vi "Longest Completion Time Job MO Swap.vi"(8 "error in (no error)":errorcluster, 9 "Schedule in":u16[](array[numeric]), 10 "OSSP_Problem":refnum<class "OSSP_Problem.lvclass">, 11 "GA in":refnum<class "GA.lvclass">) -> (0 "error out":errorcluster, 1 "Schedule out":u16[](array[numeric]), 2 "OSSP_Problem out":refnum<class "OSSP_Problem.lvclass">, 3 "GA out":refnum<class "GA.lvclass">)   [LabVIEW 2013, in "GA.lvclass"]
uses:
  GA.lvclass
  OSSP_Problem.lvclass
  GA.lvclass/GA.ctl
  OSSP_Problem.lvclass/OSSP_Problem.ctl
  Scheduler_Class/Operation to Machine Job Tuple.vi
  Scheduler_Class/Check Other Machines for Schedule Time.vi
  Scheduler_Class/Schedule Job.vi
  Scheduler_Class/Find Gaps on Particular Machine.vi
  Scheduler_Class/Increment Number of Jobs on Machine.vi
  Scheduler_Class/Find Job On Other Machines.vi
  Scheduler_Class/Prins FIFO Scheduler Methods and Controls/Methods/UpdateMachineGaps.vi
  Scheduler_Class/Prins FIFO Scheduler Methods and Controls/Methods/UpdateJobGaps.vi
  Scheduler_Class/Prins FIFO Scheduler Methods and Controls/Methods/Find Intersecting Gaps.vi
  Scheduler_Class/GT Algorithm Find M_ok and J_ok.vi
  Scheduler_Class/Prins FIFO Scheduler Methods and Controls/Methods/Transform to Plain Job and Machine Gaps Array.vi
  Scheduler.lvclass
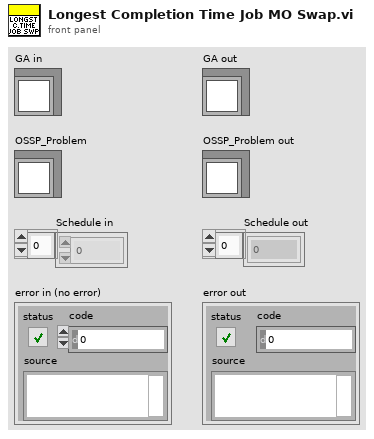
[diagram p1: front panel]
types:
  T1 = typedef "Objective.ctl" = enum16{"Makespan", "Total Tardiness"}
  T2 = typedef "Scheduler Type.ctl" = enum16{"Non Delay Scheduler", "GT Active Scheduler", "My Faulty Scheduler", "Prins FIFO Scheduler", "SemiActive Scheduler"}
  T3 = typedef "GanntChart_Element.ctl" = cluster{"Operation Number":i32, "Job Number":i32, "Start Time":i32, "Procesing Time":u16, "End Time":i32}
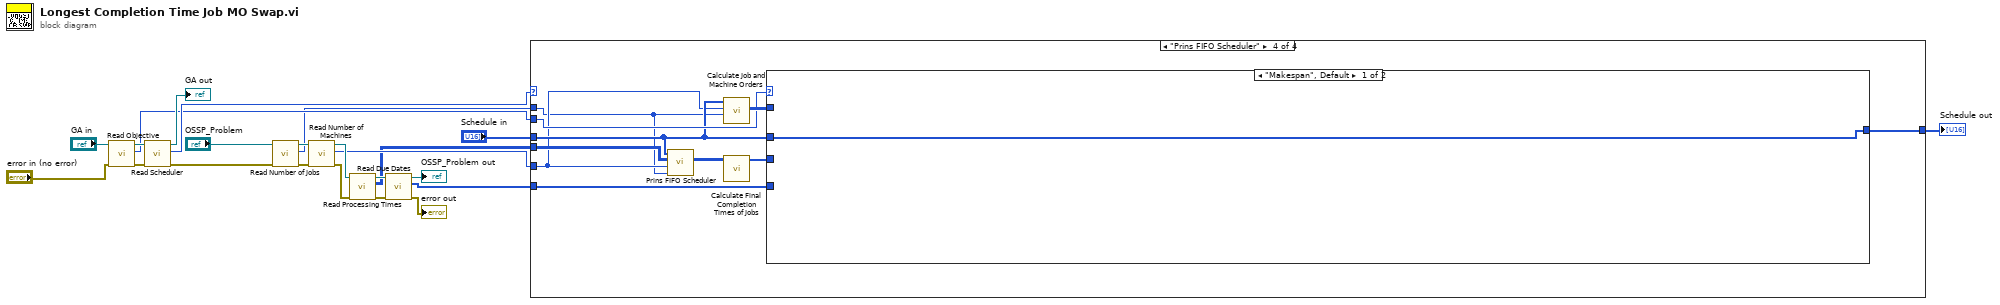
[diagram p0: block diagram]
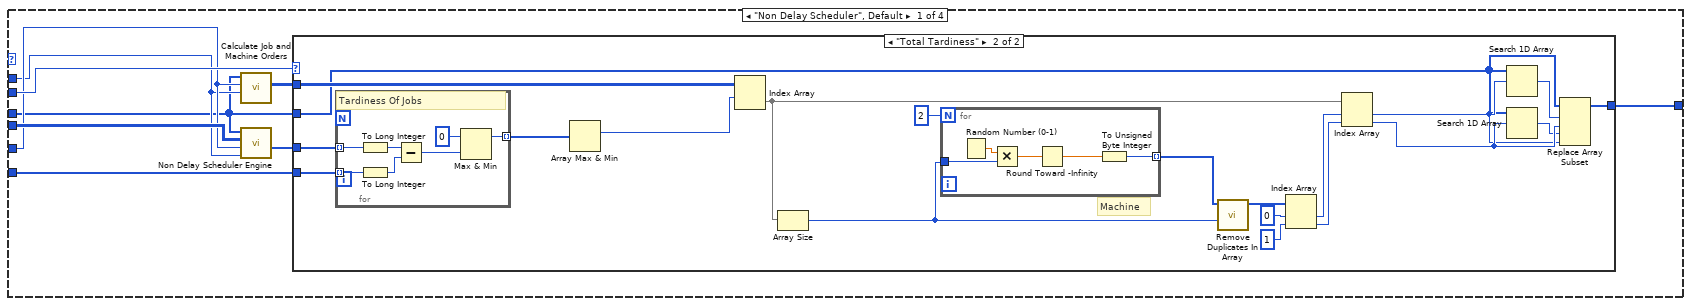
[diagram p2: hidden frame]
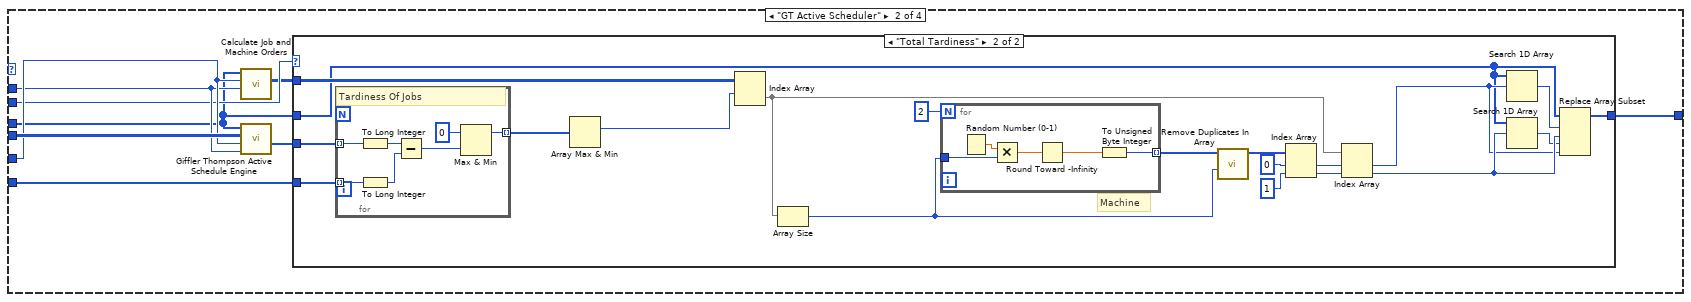
[diagram p4: hidden frame]
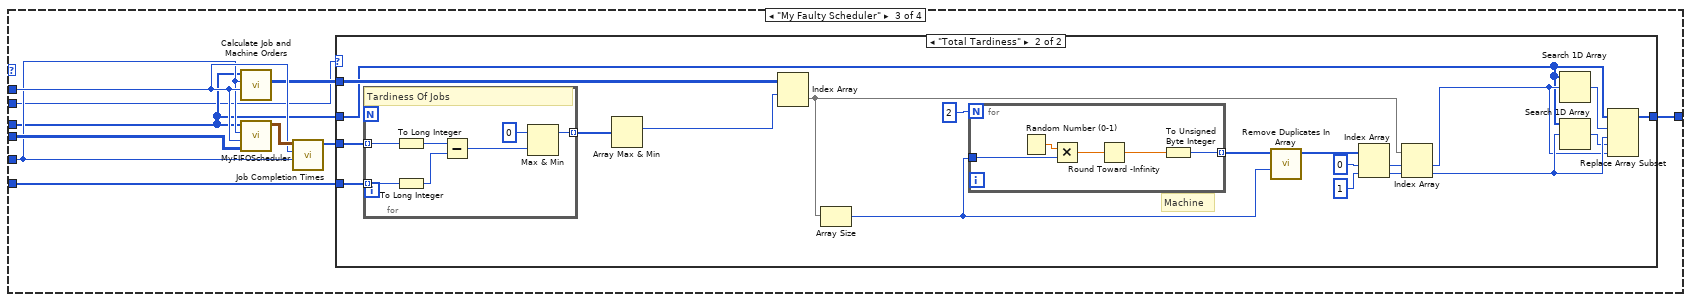
[diagram p6: hidden frame]
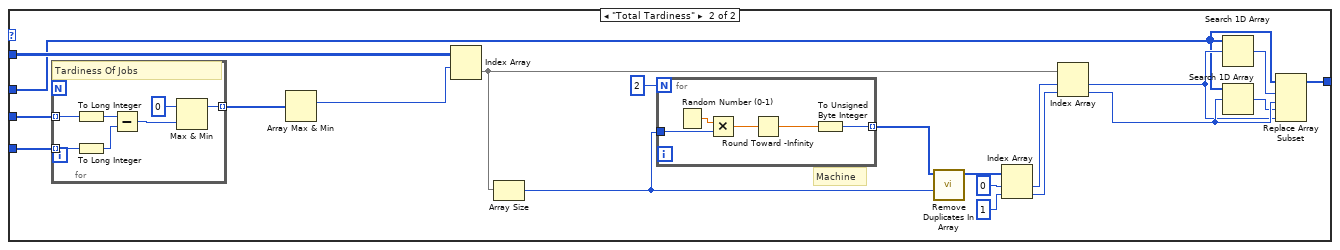
[diagram p8: hidden frame]
diagram:
  n1 = call "Read Objective .vi"("error in (no error)"="error in (no error)", "GA in"="GA in") -> ("error out"=w14:errorcluster, "Objective"=w12:T1, "GA out"=w15:refnum<class "GA.lvclass">)  [unwired: 7 in]
  n2 = call "Read Scheduler.vi"("error in (no error)"=w14, "GA in"=w15) -> ("error out"=w5:errorcluster, "Scheduler"=w13:T2, "GA out"=→"GA out":refnum<class "GA.lvclass">)  [unwired: 7 in]
  n3 = call "Read Number of Jobs.vi"("error in (no error)"=w5, "OSSP_Problem in"="OSSP_Problem") -> ("error out"=w8:errorcluster, "Number of Jobs"=w4:i32, "OSSP_Problem out"=w11:refnum<class "OSSP_Problem.lvclass">)  [unwired: 7 in]
  n4 = call "Read Number of Machines.vi"("error in (no error)"=w8, "OSSP_Problem in"=w11) -> ("error out"=w7:errorcluster, "Number of Machines"=w3:i32, "OSSP_Problem out"=w10:refnum<class "OSSP_Problem.lvclass">)  [unwired: 7 in]
  n5 = call "Read Processing Times.vi"("error in (no error)"=w7, "OSSP_Problem in"=w10) -> ("error out"=w6:errorcluster, "Processing Times"=w2:u16[][], "OSSP_Problem out"=w9:refnum<class "OSSP_Problem.lvclass">)  [unwired: 7 in]
  n6 = call "Read Due Dates.vi"("error in (no error)"=w6, "OSSP_Problem in"=w9) -> ("error out"=→"error out":errorcluster, "Due Dates"=w1:u16[], "OSSP_Problem out"=→"OSSP_Problem out":refnum<class "OSSP_Problem.lvclass">)  [unwired: 7 in]
  n7 = case shown="\"Prins FIFO Scheduler\"" w13 {
    tunnel: w12 -> [w32 w69 w108 w157]
    tunnel: w4 -> [w28 w72 w115 w153]
    tunnel: w3 -> [w29 w73 w114 w154]
    tunnel: w2 -> [w31 w74 w116 w155]
    tunnel: w1 -> [w26 w70 w112 w160]
    tunnel: "Schedule in" -> [w25 w66 w110 w156]
    tunnel: [w24 w67 w109 w158] -> w23
    frame "Non Delay Scheduler", Default {
      n8 = call "Calculate Job and Machine Orders.vi"("Number of Jobs"=w28, "Number of Machines"=w29, "Schedule"=w25) -> ("MO4J"=w27:u16[][])  [unwired: 7 in, 1 out]
      n9 = call "Non Delay Scheduler Engine.vi"("Number of  Jobs"=w28, "Number of Machines"=w29, "Processing Times"=w31, "Schedule"=w25) -> ("Job Completion Times"=w30:u16[])  [unwired: 2 in, 5 out]
      n10 = case shown="\"Total Tardiness\"" w32 {
        tunnel: w30 -> [_ w53]
        tunnel: w27 -> [_ w50]
        tunnel: w26 -> [_ w52]
        tunnel: w25 -> [w33 w35]
        tunnel: [w33 w34] -> w24
        frame "Makespan", Default {
        }
        frame "Total Tardiness" {
          # "Machine"
          n11 = for {
            tunnel: w53 -> [w65] mode=indexing
            tunnel: w52 -> [w64] mode=indexing
            tunnel: [w59] -> w51 mode=indexing
            # "Tardiness Of Jobs"
            n12 = To Long Integer(number=w65) -> (32bit integer=w63:i32)
            n13 = To Long Integer(number=w64) -> (32bit integer=w62:i32)
            n14 = Subtract(x=w63, y=w62) -> (x-y=w61:i32)
            n15 = Max & Min(x=0, y=w61) -> (max(x,y)=w59:i32)  [unwired: 1 out]
          }
          n16 = Array Max & Min(array=w51) -> (max index (indices)=w49:i32)  [unwired: 3 out]
          n17 = Index Array(array=w50, index (row)=w49) -> (element=w37:u16[])  [unwired: 1 in]
          n18 = Array Size(array=w37) -> (size(s)=w38:i32)
          n19 = for {
            N: 2 -> [_]
            tunnel: w38 -> [w57]
            tunnel: [w54] -> w41 mode=indexing
            n20 = Random Number (0-1)() -> (number: 0 to 1=w58:dbl)
            n21 = Multiply(x=w58, y=w57) -> (x*y=w56:dbl)
            n22 = Round Toward -Infinity(1:w56) -> (0:w55:dbl)
            n23 = To Unsigned Byte Integer(number=w55) -> (unsigned 8bit integer=w54:u8)
          }
          n24 = call "Remove Duplicates In Array.vi"("Max Index Bound"=w38, "Random Numbers Array"=w41) -> ("Random Numbers Array without Duplicates"=w39:i32[])  [unwired: 9 in]
          n25 = Index Array(array=w39, index #1=0 ("index"), index #2=1 ("index")) -> (element #1=w46:i32, element #2=w45:i32)
          n26 = Index Array(array=w37, index #1=w46, index #2=w45) -> (element #1=w36:u16, element #2=w43:u16)
          n27 = Search 1D Array(1D array=w35, element=w36) -> (index of element=w44:i32)  [unwired: 1 in]
          n28 = Search 1D Array(1D array=w35, element=w43) -> (index of element=w42:i32)  [unwired: 1 in]
          n29 = Replace Array Subset(array=w35, new element #1=w43, index #1=w44, new element #2=w36, index #2=w42) -> (w34:u16[])
        }
      }
    }
    frame "GT Active Scheduler" {
      n30 = call "Calculate Job and Machine Orders.vi"("Number of Jobs"=w72, "Number of Machines"=w73, "Schedule"=w66) -> ("MO4J"=w68:u16[][])  [unwired: 7 in, 1 out]
      n31 = call "Giffler Thompson Active Schedule Engine.vi"("Number of  Jobs"=w72, "Number of Machines"=w73, "Processing Times"=w74, "Schedule In"=w66) -> ("Job Completion Times"=w71:u16[])  [unwired: 3 in, 4 out]
      n32 = case shown="\"Total Tardiness\"" w69 {
        tunnel: w71 -> [_ w95]
        tunnel: w68 -> [_ w92]
        tunnel: w70 -> [_ w94]
        tunnel: w66 -> [w75 w77]
        tunnel: [w75 w76] -> w67
        frame "Makespan", Default {
        }
        frame "Total Tardiness" {
          # "Machine"
          n33 = for {
            tunnel: w95 -> [w107] mode=indexing
            tunnel: w94 -> [w106] mode=indexing
            tunnel: [w101] -> w93 mode=indexing
            # "Tardiness Of Jobs"
            n34 = To Long Integer(number=w107) -> (32bit integer=w105:i32)
            n35 = To Long Integer(number=w106) -> (32bit integer=w104:i32)
            n36 = Subtract(x=w105, y=w104) -> (x-y=w103:i32)
            n37 = Max & Min(x=0, y=w103) -> (max(x,y)=w101:i32)  [unwired: 1 out]
          }
          n38 = Array Max & Min(array=w93) -> (max index (indices)=w91:i32)  [unwired: 3 out]
          n39 = Index Array(array=w92, index (row)=w91) -> (element=w79:u16[])  [unwired: 1 in]
          n40 = Array Size(array=w79) -> (size(s)=w80:i32)
          n41 = for {
            N: 2 -> [_]
            tunnel: w80 -> [w99]
            tunnel: [w96] -> w83 mode=indexing
            n42 = Random Number (0-1)() -> (number: 0 to 1=w100:dbl)
            n43 = Multiply(x=w100, y=w99) -> (x*y=w98:dbl)
            n44 = Round Toward -Infinity(1:w98) -> (0:w97:dbl)
            n45 = To Unsigned Byte Integer(number=w97) -> (unsigned 8bit integer=w96:u8)
          }
          n46 = call "Remove Duplicates In Array.vi"("Max Index Bound"=w80, "Random Numbers Array"=w83) -> ("Random Numbers Array without Duplicates"=w81:i32[])  [unwired: 9 in]
          n47 = Index Array(array=w81, index #1=0 ("index"), index #2=1 ("index")) -> (element #1=w88:i32, element #2=w87:i32)
          n48 = Index Array(array=w79, index #1=w88, index #2=w87) -> (element #1=w78:u16, element #2=w85:u16)
          n49 = Search 1D Array(1D array=w77, element=w78) -> (index of element=w86:i32)  [unwired: 1 in]
          n50 = Search 1D Array(1D array=w77, element=w85) -> (index of element=w84:i32)  [unwired: 1 in]
          n51 = Replace Array Subset(array=w77, new element #1=w85, index #1=w86, new element #2=w78, index #2=w84) -> (w76:u16[])
        }
      }
    }
    frame "My Faulty Scheduler" {
      n52 = call "Calculate Job and Machine Orders.vi"("Number of Jobs"=w115, "Number of Machines"=w114, "Schedule"=w110) -> ("MO4J"=w111:u16[][])  [unwired: 7 in, 1 out]
      n53 = call "MyFIFOScheduler.vi"("Processing Times (Rows Mach.Cols Jobs)"=w116, "Number of Jobs"=w115, "Number of Machines"=w114, "Schedule"=w110) -> ("Gannt Chart Out"=w117:T3[][])  [unwired: 6 in, 1 out]
      n54 = call "Job Completion Times.vi"("Number Of Machines"=w114, "Number Of Jobs"=w115, "Gannt Chart In"=w117) -> ("Job Completion Times"=w113:u16[])  [unwired: 8 in]
      n55 = case shown="\"Total Tardiness\"" w108 {
        tunnel: w113 -> [_ w138]
        tunnel: w111 -> [_ w135]
        tunnel: w112 -> [_ w137]
        tunnel: w110 -> [w118 w120]
        tunnel: [w118 w119] -> w109
        frame "Makespan", Default {
        }
        frame "Total Tardiness" {
          # "Machine"
          n56 = for {
            tunnel: w138 -> [w150] mode=indexing
            tunnel: w137 -> [w149] mode=indexing
            tunnel: [w144] -> w136 mode=indexing
            # "Tardiness Of Jobs"
            n57 = To Long Integer(number=w150) -> (32bit integer=w148:i32)
            n58 = To Long Integer(number=w149) -> (32bit integer=w147:i32)
            n59 = Subtract(x=w148, y=w147) -> (x-y=w146:i32)
            n60 = Max & Min(x=0, y=w146) -> (max(x,y)=w144:i32)  [unwired: 1 out]
          }
          n61 = Array Max & Min(array=w136) -> (max index (indices)=w134:i32)  [unwired: 3 out]
          n62 = Index Array(array=w135, index (row)=w134) -> (element=w122:u16[])  [unwired: 1 in]
          n63 = Array Size(array=w122) -> (size(s)=w123:i32)
          n64 = for {
            N: 2 -> [_]
            tunnel: w123 -> [w142]
            tunnel: [w139] -> w126 mode=indexing
            n65 = Random Number (0-1)() -> (number: 0 to 1=w143:dbl)
            n66 = Multiply(x=w143, y=w142) -> (x*y=w141:dbl)
            n67 = Round Toward -Infinity(1:w141) -> (0:w140:dbl)
            n68 = To Unsigned Byte Integer(number=w140) -> (unsigned 8bit integer=w139:u8)
          }
          n69 = call "Remove Duplicates In Array.vi"("Max Index Bound"=w123, "Random Numbers Array"=w126) -> ("Random Numbers Array without Duplicates"=w124:i32[])  [unwired: 9 in]
          n70 = Index Array(array=w124, index #1=0 ("index"), index #2=1 ("index")) -> (element #1=w131:i32, element #2=w130:i32)
          n71 = Index Array(array=w122, index #1=w131, index #2=w130) -> (element #1=w121:u16, element #2=w128:u16)
          n72 = Search 1D Array(1D array=w120, element=w121) -> (index of element=w129:i32)  [unwired: 1 in]
          n73 = Search 1D Array(1D array=w120, element=w128) -> (index of element=w127:i32)  [unwired: 1 in]
          n74 = Replace Array Subset(array=w120, new element #1=w128, index #1=w129, new element #2=w121, index #2=w127) -> (w119:u16[])
        }
      }
    }
    frame "Prins FIFO Scheduler" {
      n75 = call "Prins FIFO Scheduler.vi"("Number of Jobs"=w153, "Number of Machines"=w154, "Processing Times(MxJ)"=w155, "Schedule In"=w156) -> ("Completion Times (MxJ)"=w152:i32[][])  [unwired: 6 in, 1 out]
      n76 = call "Calculate Job and Machine Orders.vi"("Number of Jobs"=w153, "Number of Machines"=w154, "Schedule"=w156) -> ("MO4J"=w159:u16[][])  [unwired: 7 in, 1 out]
      n77 = call "Calculate Final Completion Times of Jobs.vi"("Completion Times (MxJ)"=w152) -> ("Job Completion Times"=w151:i32[])  [unwired: 10 in]
      n78 = case shown="\"Makespan\", Default" w157 {
        tunnel: w151 -> [_ w181]
        tunnel: w159 -> [_ w178]
        tunnel: w160 -> [_ w180]
        tunnel: w156 -> [w161 w163]
        tunnel: [w161 w162] -> w158
        frame "Makespan", Default {
        }
        frame "Total Tardiness" {
          # "Machine"
          n79 = for {
            tunnel: w181 -> [w193] mode=indexing
            tunnel: w180 -> [w192] mode=indexing
            tunnel: [w187] -> w179 mode=indexing
            # "Tardiness Of Jobs"
            n80 = To Long Integer(number=w193) -> (32bit integer=w191:i32)
            n81 = To Long Integer(number=w192) -> (32bit integer=w190:i32)
            n82 = Subtract(x=w191, y=w190) -> (x-y=w189:i32)
            n83 = Max & Min(x=0, y=w189) -> (max(x,y)=w187:i32)  [unwired: 1 out]
          }
          n84 = Array Max & Min(array=w179) -> (max index (indices)=w177:i32)  [unwired: 3 out]
          n85 = Index Array(array=w178, index (row)=w177) -> (element=w165:u16[])  [unwired: 1 in]
          n86 = Array Size(array=w165) -> (size(s)=w166:i32)
          n87 = for {
            N: 2 -> [_]
            tunnel: w166 -> [w185]
            tunnel: [w182] -> w169 mode=indexing
            n88 = Random Number (0-1)() -> (number: 0 to 1=w186:dbl)
            n89 = Multiply(x=w186, y=w185) -> (x*y=w184:dbl)
            n90 = Round Toward -Infinity(1:w184) -> (0:w183:dbl)
            n91 = To Unsigned Byte Integer(number=w183) -> (unsigned 8bit integer=w182:u8)
          }
          n92 = call "Remove Duplicates In Array.vi"("Max Index Bound"=w166, "Random Numbers Array"=w169) -> ("Random Numbers Array without Duplicates"=w167:i32[])  [unwired: 9 in]
          n93 = Index Array(array=w167, index #1=0 ("index"), index #2=1 ("index")) -> (element #1=w174:i32, element #2=w173:i32)
          n94 = Index Array(array=w165, index #1=w174, index #2=w173) -> (element #1=w164:u16, element #2=w171:u16)
          n95 = Search 1D Array(1D array=w163, element=w164) -> (index of element=w172:i32)  [unwired: 1 in]
          n96 = Search 1D Array(1D array=w163, element=w171) -> (index of element=w170:i32)  [unwired: 1 in]
          n97 = Replace Array Subset(array=w163, new element #1=w171, index #1=w172, new element #2=w164, index #2=w170) -> (w162:u16[])
        }
      }
    }
  }
  "Schedule out" <- w23
